vi "To JSON.vi"(0 "Anything":variant, 1 "Pretty Print (F)":bool) -> (2 "JSON":string)   [LabVIEW 2013, in "LV JSON.lvlib"]
uses:
  LV JSON.lvlib
  <vilib>/dlg_ctls.llb/Space Constant.vi
  subVIs/JSON No Whitespace.vi
  <vilib>/Utility/error.llb/Trim Whitespace.vi
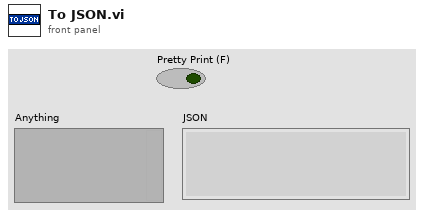
[diagram p1: front panel]
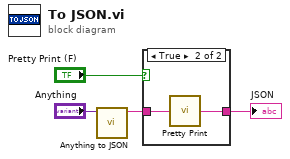
[diagram p0: block diagram]
diagram:
  n1 = call "Anything to JSON.vi"("Anything"="Anything") -> ("JSON"=w2:string)  [unwired: 8 in, 2 out]
  n2 = case shown="True" "Pretty Print (F)" {
    tunnel: w2 -> [w5 w7]
    tunnel: [w5 w6] -> w1
    frame False {
    }
    frame True {
      n3 = call "Pretty Print.vi"("JSON String"=w7) -> ("Pretty JSON String"=w6:string)  [unwired: 1 out]
    }
  }
  "JSON" <- w1
